vi "Get 1D B Array.vi"(0 "B":dbl[][](array[numeric])) -> (1 "B 1D":dbl[](array[numeric]), 2 "Nx":i32, 3 "Ny":i32)   [LabVIEW 2016]
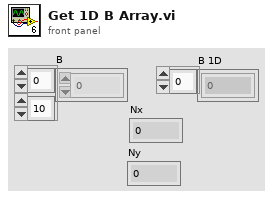
[diagram p1: front panel]
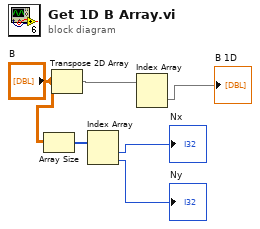
[diagram p0: block diagram]
diagram:
  n1 = Array Size(array="B") -> (size(s)=w3:i32[])
  n2 = Transpose 2D Array(2D array="B") -> (transposed array=w6:dbl[][])
  n3 = Index Array(array=w3) -> (element #1=→"Nx":i32, element #2=→"Ny":i32)  [unwired: 2 in]
  n4 = Index Array(array=w6) -> (element=→"B 1D":dbl[])  [unwired: 2 in]
